vi "ROI group-Update group name in ctrl.vi"(6 "Index of group to update":i32, 8 "error in (no error)":errorcluster, 11 "Group Name":string) -> (0 "error out":errorcluster)   [LabVIEW 2020]
uses:
  Global variables/gl_Functional Imaging-Global variables.vi
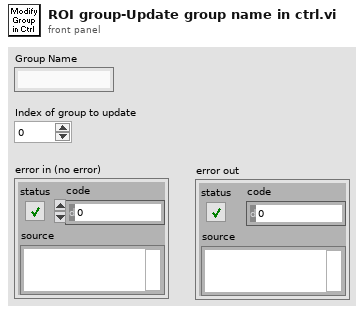
[diagram p1: front panel]
types:
  T1 = typedef "Functional Imging UI Refs.ctl" = cluster{"Menu ref":refnum<k9>, "Image control":refnum<vi>, "VI ref":refnum<vi>, "XGrapher":refnum<vi>, "Smoothing":refnum<vi>, "POI Averaging":refnum<vi>, "Normalize":refnum<vi>, "POI data points in each trial":refnum<vi>, "Channel":refnum<vi>, "Experiment data folder path":refnum<vi>, "[ROI vis]":refnum<vi>, "[Groups] visbl":T2, "Group Name":refnum<vi>, "POI index":refnum<vi>, "Trial No.":refnum<vi>, "Intensity Zoom":refnum<vi>, "Trial Cursor Enabled":refnum<vi>, "Number of Trials (ind 1)":refnum<vi>, "Number of Trials (ind 2)":refnum<vi>, "MiniScans Available":refnum<vi>, "POI Available":refnum<vi>, "Defer graph updates":refnum<vi>, "Waveform selector":refnum<vi>, "#of selected POI":refnum<vi>, "#of selected MiniScans":refnum<vi>, "#of selected groups":refnum<vi>, "Max Z-Projection":refnum<vi>, "Z-Plane Selector":refnum<vi>, "Index of miniscan point to visualise":refnum<vi>, "ROI vis. mode":refnum<vi>, "Total # of points":refnum<vi>, "Index of group clicked on":refnum<vi>, "Pane 1":refnum<vi>, "Pane 2":refnum<vi>, "Pane 3":refnum<vi>, "Pane 4":refnum<vi>, "Pane 5":refnum<vi>, "Pane 6":refnum<vi>, "Deselect all ROI":refnum<vi>, "Deselect all groups":refnum<vi>}
  T2 = typedef "Groups array referecne.ctl" = refnum<vi>
  T3 = typedef "Group sel cluster.ctl" = cluster{"Group number":string, "Group Name":string, "Visibility":bool, "Highlight":bool}
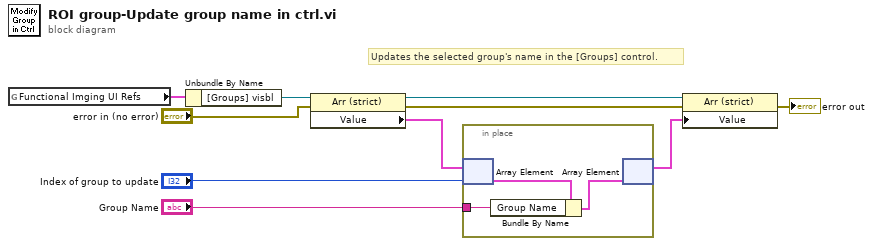
[diagram p0: block diagram]
diagram:
  # "Updates the selected group's name in the [Groups] control."
  n1 = global read "gl_Functional Imaging-Global variables.vi" "Functional Imging UI Refs"() -> (w2:T1)
  n2 = Unbundle By Name(w2) -> ("[Groups] visbl"=w9:T2)
  n3 = property on="Property Node" class="Arr (strict)"(reference=w9, error in="error in (no error)") -> (reference out=w10:T2, error out=w7:errorcluster, "Value"=w6:T3[])
  n4 = in-place {
    in-place-border: "Group Name" -> [w11]
    n5 = in-place-array #1(w6, "Index of group to update") -> (w13:T3)
    n6 = Bundle By Name(cluster=w13, "Group Name"=w11) -> (w12:T3)
    n7 = in-place-array #1(w12) -> (w5:T3[])  [unwired: 1 out]
  }
  n8 = property on="Property Node" class="Arr (strict)"(reference=w10, error in=w7, "Value"=w5) -> (error out=→"error out":errorcluster)  [unwired: 1 out]
